vi "UART Read Data.vi"(7 "UART #":T1=-1, 8 "error in (no error)":errorcluster, 9 "Len (LineTerm)":u8, 11 "Session in":refnum<class "Session.lvclass">) -> (0 "error out":errorcluster, 1 "Data":string, 3 "Session out":refnum<class "Session.lvclass">)   [LabVIEW 2024, in "CTI.lvlib" / "Session.lvclass"]
doc: "Reads data from a UART connection. If Len is set to a non-default value, the device will attempt to read the specified number of bytes from the UART port. If Len is left as its default value, the UART will finish reading as soon as the configured line term character/byte has been read."
uses:
  Session.lvclass
  UART Number.ctl
  DeviceComms/DeviceComms.lvclass
  CTI.lvlib
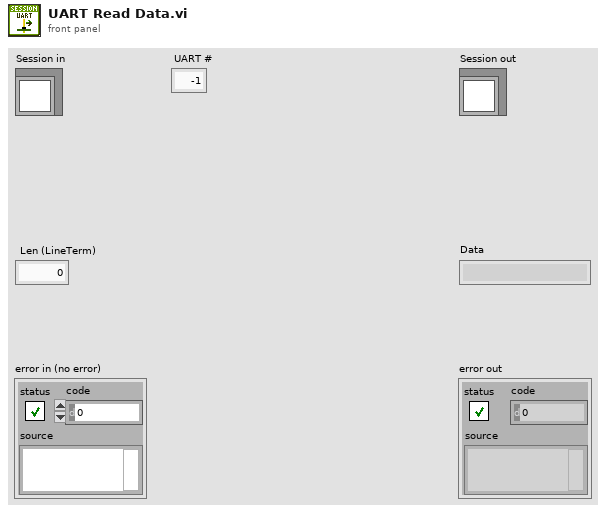
[diagram p1: front panel]
types:
  T1 = typedef "CTI.lvlib/UART Number.ctl" = i8
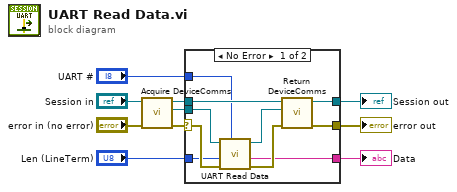
[diagram p0: block diagram]
diagram:
  n1 = call "Acquire DeviceComms.vi"("error in (no error)"="error in (no error)", "Session in"="Session in") -> ("error out"=w9:errorcluster, "DeviceComms"=w8:refnum<class "DeviceComms.lvclass">, "Session out"=w10:refnum<class "Session.lvclass">)  [unwired: 7 in]
  n2 = case shown="No Error" w9 {
    selector: w9 -> [w19 w22]
    tunnel: w10 -> [w18 w21]
    tunnel: w8 -> [w20 _]
    tunnel: [w15 w21] -> w2
    tunnel: [w14 w22] -> w1
    tunnel: "UART #" -> [w13 _]
    tunnel: "Len (LineTerm)" -> [w12 _]
    tunnel: [w11 _] -> w3
    frame No Error {
      n3 = call-dynamic "UART Read Data.vi"("UART #"=w13, "error in (no error)"=w19, "Len (LineTerm)"=w12, "DeviceComms in"=w20) -> ("error out"=w16:errorcluster, "Data"=w11:string, "DeviceComms out"=w17:refnum<class "DeviceComms.lvclass">)  [unwired: 5 in]
      n4 = call "Return DeviceComms.vi"("error in (no error)"=w16, "DeviceComms"=w17, "Session in"=w18) -> ("error out"=w14:errorcluster, "Session out"=w15:refnum<class "Session.lvclass">)  [unwired: 7 in]
    }
    frame Error {
    }
  }
  "error out" <- w1
  "Session out" <- w2
  "Data" <- w3
